vi "get.vol.id.vi"(7 "map in":map{i32, path}(c390), 8 "error in (no error)":errorcluster, 11 "Path":path) -> (0 "error out":errorcluster, 1 "volume":i32, 2 "volume type":T1 caption="Enum", 3 "id":i32)   [LabVIEW 2024, in "CV_downloader.lvclass"]
uses:
  CV_downloader.lvclass
  CV_Shared_Library/volume.type--enum.ctl
  <userlib>/_OpenG.lib/file/file.llb/Strip Path Extension - String__ogtk.vi
  <userlib>/_OpenG.lib/file/file.llb/openg_file.lvlib
  CV_Shared_Library/CV_Shared_Library.lvlib
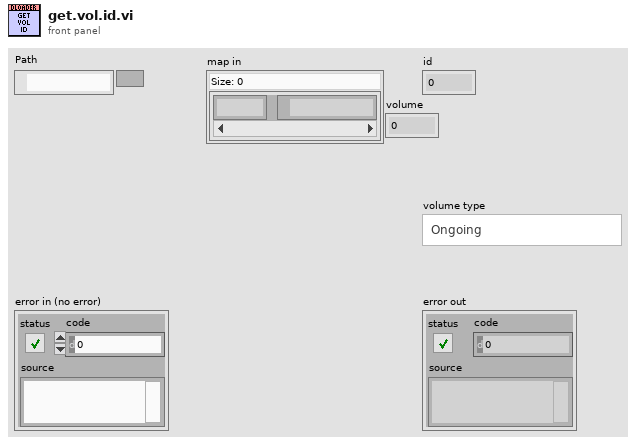
[diagram p1: front panel]
types:
  T1 = typedef "CV_Shared_Library.lvlib/volume.type--enum.ctl" = enum16{"Ongoing", "Limited Series", "Annual", "One Shot", "Reprint/Document", "Star Comics", "Epic Comics"}
  T2 = typedef "CV_RESTful_Lib.lvlib/local_volume--cluster.ctl" = cluster{"id":i32, "name":string, "sortable_name":string, "aliases":string[], "description":string, "site_detail_url":string, "count_of_issues":i32, "start_year":i32, "publisher_id":i32, "issue_ids":i32[], "date_last_updated":timestamp, "volume":i32, "cv_id":string, "volume type":T1}
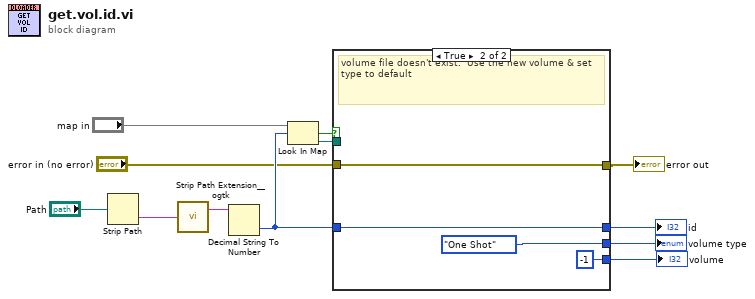
[diagram p0: block diagram]
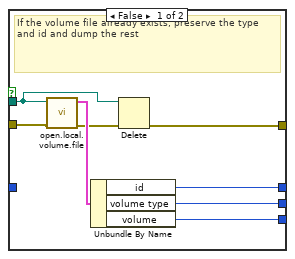
[diagram p2: hidden frame]
diagram:
  n1 = Strip Path(path="Path") -> (name=w10:string)  [unwired: 1 out]
  n2 = call-poly <userlib>:"Strip Path Extension__ogtk.vi"("path"=w10) -> ("root"=w9:string)  [unwired: 1 out]
  n3 = Decimal String To Number(string=w9) -> (number=w6:i32)  [unwired: 2 in, 1 out]
  n4 = Look In Map(map="map in", key=w6) -> (key not found?=w8:bool, value=w7:path)  [unwired: 1 in]
  n5 = case shown="True" w8 {
    tunnel: w7 -> [w16 _]
    tunnel: [w19 w24] -> w4
    tunnel: w6 -> [_ w24]
    tunnel: [w18 volume.type--enum."One Shot" ("volume type")] -> w5
    tunnel: [w15 w22] -> w3
    tunnel: "error in (no error)" -> [w14 w22]
    tunnel: [w13 -1 ("volume")] -> w1
    frame False {
      # "If the volume file already exists, preserve the type and id and dump the rest"
      n6 = call "open.local.volume.file.vi"("error in (no error)"=w14, "volume json"=w16) -> ("error out"=w17:errorcluster, "volume"=w20:T2)  [unwired: 8 in]
      n7 = Unbundle By Name(w20) -> ("id"=w19:i32, "volume type"=w18:T1, "volume"=w13:i32)
      n8 = Delete(path (use dialog)=w16, error in=w17) -> (error out=w15:errorcluster)  [unwired: 3 in, 2 out]
    }
    frame True {
      # "volume file doesn't exist.  Use the new volume & set type to default"
    }
  }
  "volume type" <- w5
  "id" <- w4
  "error out" <- w3
  "volume" <- w1
